vi "hasPacketIdentifier.vi"(11 "PUBACK in":refnum<class "PUBACK.lvclass">) -> (2 "Has Packet Identifier":bool, 3 "PUBACK out":refnum<class "PUBACK.lvclass">)   [LabVIEW 2013, in "MQTT_Control_Packets.lvlib" / "PUBACK.lvclass"]
uses:
  PUBACK.lvclass
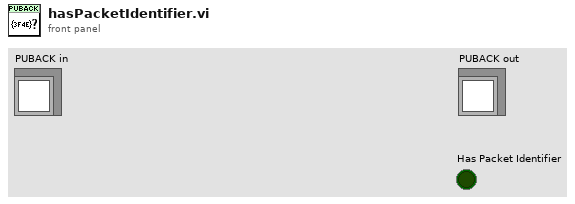
[diagram p1: front panel]
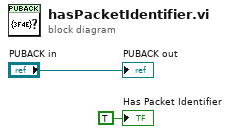
[diagram p0: block diagram]
diagram:
  "PUBACK out" <- "PUBACK in"
  "Has Packet Identifier" <- TRUE ("As Packet Identifier")
